vi "ActionVIOnLoad.vi"(8 "error in (no error)":errorcluster, 11 "Device Item Ref in":T1 format="%.0x") -> (0 "error out":errorcluster, 3 "Device Item Ref out":T1 format="%.0x")   [LabVIEW 2019, in "Protection and Counter Addon System Explorer.lvlib"]
uses:
  Protection and Counter Addon System Explorer.lvlib
  <vilib>/NI VeriStand/Custom Device API/Custom Device Item Ref.ctl
  <vilib>/NI VeriStand/Custom Device API/Custom Device Channel.ctl
  <vilib>/NI VeriStand/Custom Device API/Custom Device Channel Type.ctl
  NationalInstruments.VeriStand.SystemDefinitionAPI
  Addon Shared/SubVIs/GUID Lookup.vi
  <vilib>/NI/NI VeriStand Advanced SysDef API/_SubVIs/SysDef.Search.GUID.vi
  <vilib>/NI/NI VeriStand Advanced SysDef API/_SubVIs/SysDef.Search.GUIDs.vi
  <vilib>/NI/NI VeriStand Advanced SysDef API/_SubVIs/SysDef.Search.Parent.vi
  Addon Shared/Protection and Counter Addon Shared.lvlib
  <vilib>/NI/NI VeriStand Advanced SysDef API/SysDef API/Advanced System Definition.lvlib
  <vilib>/NI VeriStand/Custom Device API/Custom Device API.lvlib
  SubModules/Frame-Protection-Support/Source/System Explorer/Protection and Counter Support System Explorer.lvlib
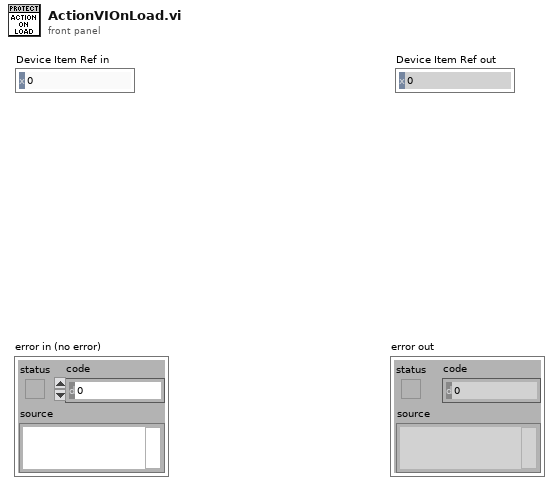
[diagram p1: front panel]
types:
  T1 = typedef "Custom Device API.lvlib/Custom Device Item Ref.ctl" = u64
  T2 = typedef "Custom Device API.lvlib/Custom Device Channel.ctl" = cluster{"Type":T3, "Units":string, "Default Value":dbl, "Faultable":bool, "Scalable":bool}
  T3 = typedef "Custom Device API.lvlib/Custom Device Channel Type.ctl" = enum16{"Input", "Output"}
  T4 = typedef "Protection and Counter Support System Explorer.lvlib/Protection Signal Settings.ctl" = cluster{"Input Channels":T5[], "Protection Type":T6}
  T5 = typedef "Protection and Counter Support System Explorer.lvlib/Protection Signal Linked Channel.ctl" = cluster{"Node Ref":T1}
  T6 = typedef "Protection and Counter Support Shared.lvlib/Protection Type.ctl" = enum16{"Arb ID + Bytes Checksum with Inversion", "Arb ID + Bytes CRC with Inversion", "Reversed Raw Signal Checksum with Inversion", "Concatenated Two's Compliment"}
  T7 = typedef "Advanced System Definition.lvlib/TreeItem.Info.ctl" = cluster{"Name":string, "Description":string, "GUID":string, "Is Channel":bool, "Channel":T2, "Is Waveform":bool, "Waveform":T8}
  T8 = typedef "Custom Device API.lvlib/Custom Device Waveform.ctl" = cluster{"Data Type":T9, "Units":string}
  T9 = typedef "Custom Device API.lvlib/Custom Device Waveform DataType.ctl" = enum16{"Double", "Complex Double"}
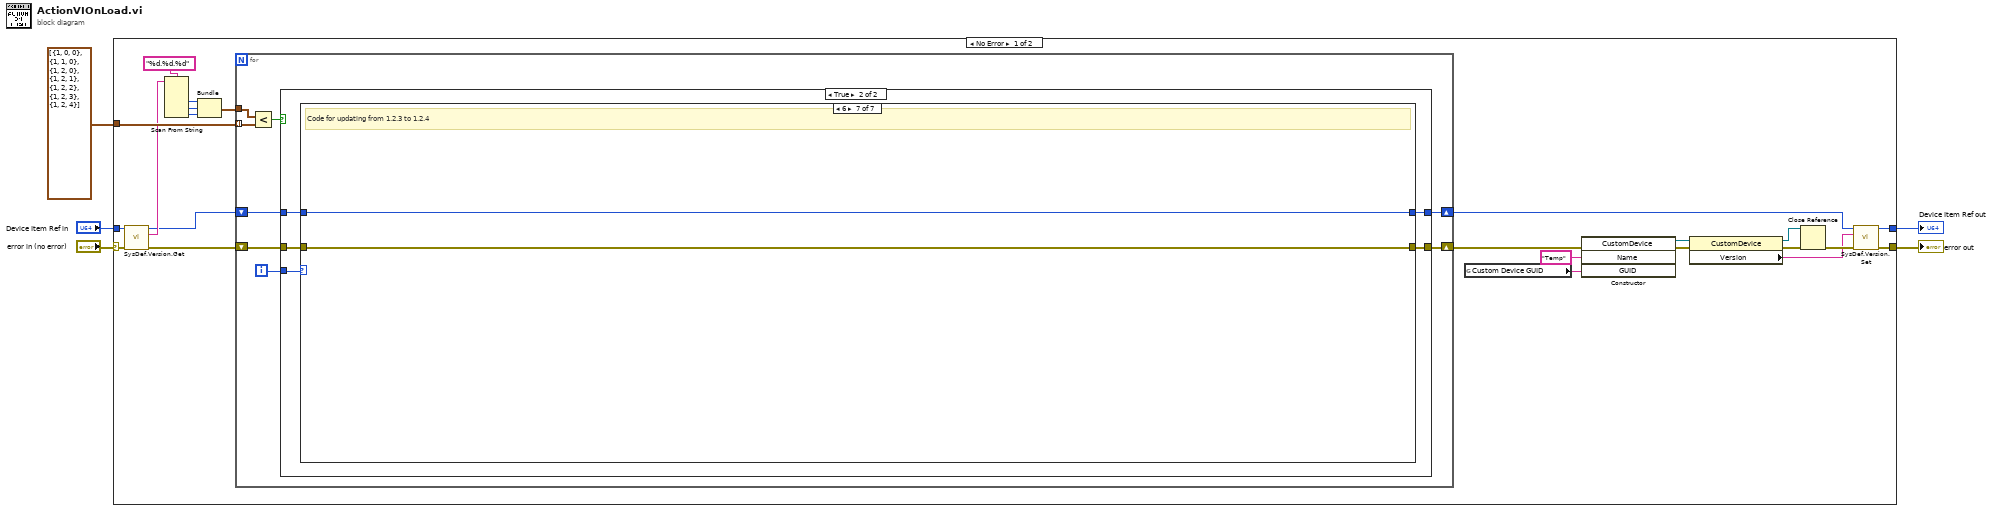
[diagram p0: block diagram]
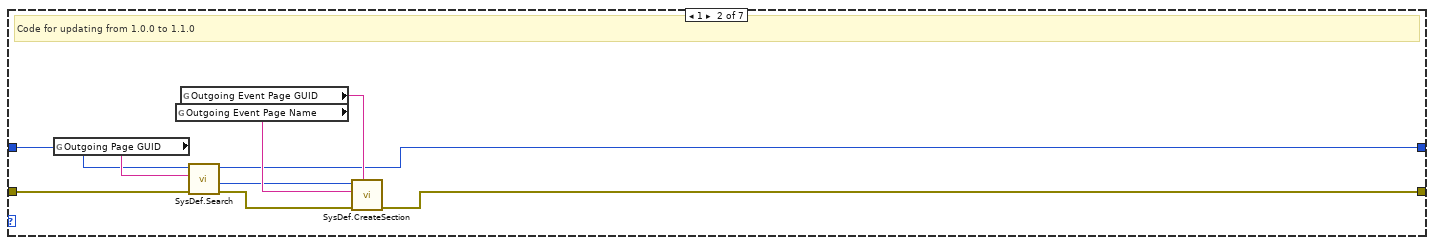
[diagram p4: hidden frame]
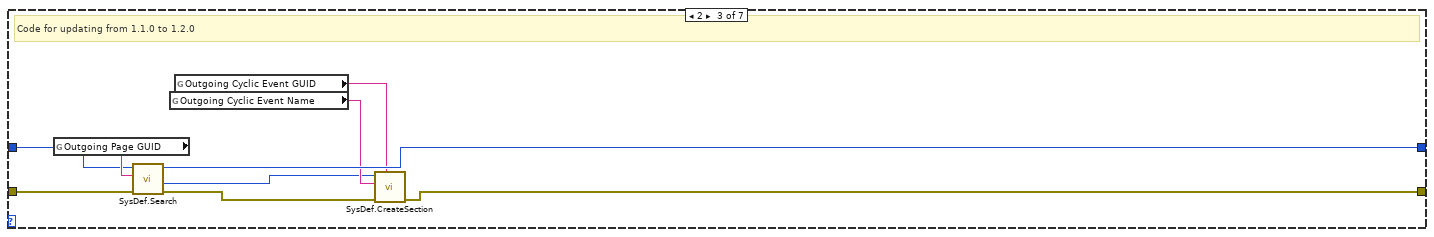
[diagram p5: hidden frame]
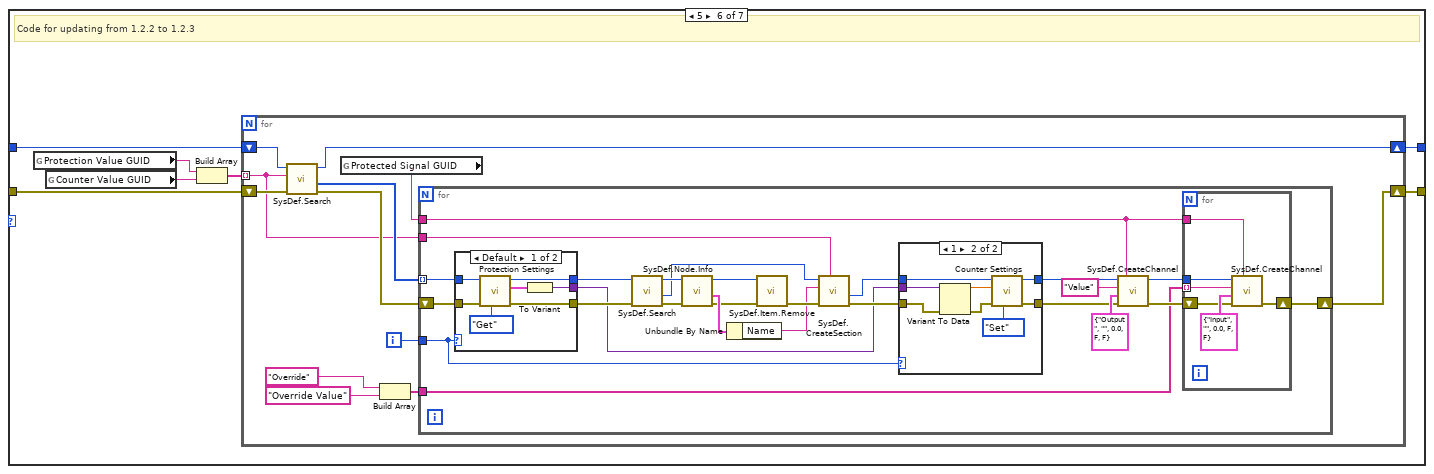
[diagram p8: hidden frame]
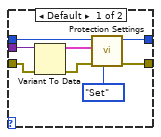
[diagram p9: hidden frame]
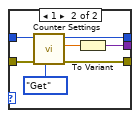
[diagram p10: hidden frame]
diagram:
  n1 = case shown="No Error" "error in (no error)" {
    selector: "error in (no error)" -> [w11 w152]
    tunnel: [w18 w152] -> w4
    tunnel: "Device Item Ref in" -> [w10 w151]
    tunnel: [w16 w151] -> w2
    tunnel: cluster{i32, i32, i32}[] [{1, 0, 0}, {1, 1, 0}, {1, 2, 0}, {1, 2, 1}, {1, 2, 2}, {1, 2, 3}, {1, 2, 4}] -> [w20 _]
    frame No Error {
      n2 = call <vilib>:"SysDef.Version.Get.vi"("error in (no error)"=w11, "nodeID"=w10) -> ("error out"=w7:errorcluster, "Version"=w14:string, "nodeID out"=w6:u64)  [unwired: 7 in]
      n3 = Scan From String(format string="%d.%d.%d", input string=w14) -> (output 1=w13:i32, output 2=w12:i32, output 3=w15:i32)  [unwired: 5 in, 3 out]
      n4 = Bundle(w13, w12, w15) -> (w8:cluster{i32, i32, i32})  [unwired: 1 in]
      n5 = for {
        tunnel: w20 -> [w31] mode=indexing
        shift-right: [w35] -> w19
        shift-left: w7 -> [w29]
        shift-right: [w34] -> w21
        shift-left: w6 -> [w30]
        tunnel: w8 -> [w32]
        i -> [w33]
        n6 = Less?(x=w32, y=w31) -> (x < y?=w36:bool)
        n7 = case shown="True" w36 {
          tunnel: w29 -> [w38 w43]
          tunnel: w30 -> [w37 w42]
          tunnel: [w38 w40] -> w35
          tunnel: [w37 w41] -> w34
          tunnel: w33 -> [_ w39]
          frame False {
          }
          frame True {
            n8 = case shown="6" w39 {
              tunnel: w43 -> [w44 w51 w62 w64 w66 w73 w149]
              tunnel: w42 -> [w45 w50 w61 w65 w67 w68 w150]
              tunnel: [w45 w47 w60 w65 w67 w74 w150] -> w41
              tunnel: [w44 w46 w57 w64 w66 w72 w149] -> w40
              frame Default {
              }
              frame 1 {
                # "Code for updating from 1.0.0 to 1.1.0"
                n9 = global read "GUID Lookup.vi" "Outgoing Page GUID"() -> (w52:string)
                n10 = global read "GUID Lookup.vi" "Outgoing Event Page Name"() -> (w54:string)
                n11 = global read "GUID Lookup.vi" "Outgoing Event Page GUID"() -> (w53:string)
                n12 = call-poly <vilib>:"SysDef.Search.vi"("error in (no error)"=w51, "GUID"=w52, "nodeID"=w50) -> ("error out"=w49:errorcluster, "Value out"=w48:u64, "nodeID out"=w47:u64)  [unwired: 5 in, 1 out]
                n13 = call <vilib>:"SysDef.CreateSection.vi"("GUID"=w53, "error in (no error)"=w49, "Name"=w54, "nodeID"=w48) -> ("error out"=w46:errorcluster)  [unwired: 4 in, 3 out]
              }
              frame 2 {
                # "Code for updating from 1.1.0 to 1.2.0"
                n14 = global read "GUID Lookup.vi" "Outgoing Page GUID"() -> (w63:string)
                n15 = call-poly <vilib>:"SysDef.Search.vi"("error in (no error)"=w62, "GUID"=w63, "nodeID"=w61) -> ("error out"=w56:errorcluster, "Value out"=w55:u64, "nodeID out"=w60:u64)  [unwired: 5 in, 1 out]
                n16 = global read "GUID Lookup.vi" "Outgoing Cyclic Event Name"() -> (w59:string)
                n17 = global read "GUID Lookup.vi" "Outgoing Cyclic Event GUID"() -> (w58:string)
                n18 = call <vilib>:"SysDef.CreateSection.vi"("GUID"=w58, "error in (no error)"=w56, "Name"=w59, "nodeID"=w55) -> ("error out"=w57:errorcluster)  [unwired: 4 in, 3 out]
              }
              frame 3 {
                # "Code for updating from 1.2.0 to 1.2.1"
              }
              frame 4 {
                # "Code for updating from 1.2.1 to 1.2.2"
              }
              frame 5 {
                # "Code for updating from 1.2.2 to 1.2.3"
                n19 = global read "GUID Lookup.vi" "Protection Value GUID"() -> (w71:string)
                n20 = global read "GUID Lookup.vi" "Counter Value GUID"() -> (w70:string)
                n21 = Build Array(w71, w70) -> (w69:string[])
                n22 = for {
                  shift-right: [w86] -> w74
                  shift-left: w68 -> [w85]
                  shift-right: [w81] -> w72
                  shift-left: w73 -> [w84]
                  tunnel: w69 -> [w76] mode=indexing
                  i -> [w75]
                  n23 = call-poly <vilib>:"SysDef.Search.vi"("error in (no error)"=w84, "GUID"=w76, "nodeID"=w85) -> ("error out"=w82:errorcluster, "Values Out"=w83:u64[], "nodeID out"=w86:u64)  [unwired: 5 in, 1 out]
                  n24 = global read "GUID Lookup.vi" "Protected Signal GUID"() -> (w77:string)
                  n25 = Build Array("Override" ("Override Name"), "Override Value" ("Override Value Name")) -> (w78:string[])
                  n26 = for {
                    tunnel: w83 -> [w93] mode=indexing
                    shift-right: [w110] -> w81
                    shift-left: w82 -> [w96]
                    tunnel: w78 -> [w109]
                    tunnel: w77 -> [w107]
                    tunnel: w76 -> [w100]
                    tunnel: w75 -> [w87]
                    n27 = case shown="Default" w87 {
                      tunnel: w96 -> [w133 w141]
                      tunnel: [w132 w140] -> w95
                      tunnel: [w131 w139] -> w94
                      tunnel: w93 -> [w134 w138]
                      tunnel: [w129 w136] -> w88
                      frame Default {
                        n28 = call "Protection Settings.vi"("Action"=enum8{"Get", "Set"}."Get", "error in"=w133, "Parent Ref"=w134) -> ("error out"=w132:errorcluster, "Selected Channels"=w130:T4, "Parent Ref Out"=w131:T1)  [unwired: 6 in]
                        n29 = To Variant(anything=w130) -> (Variant=w129:variant)
                      }
                      frame 1 {
                        n30 = call "Counter Settings.vi"("Action"=enum8{"Get", "Set"}."Get", "error in"=w141, "Parent Ref"=w138) -> ("error out"=w140:errorcluster, "Max Count"=w137:dbl, "Parent Ref Out"=w139:T1)  [unwired: 6 in]
                        n31 = To Variant(anything=w137) -> (Variant=w136:variant)
                      }
                    }
                    n32 = call-poly <vilib>:"SysDef.Search.vi"("error in (no error)"=w95, "nodeID"=w94) -> ("error out"=w99:errorcluster, "Value out"=w97:u64, "nodeID out"=w98:u64)  [unwired: 6 in, 1 out]
                    n33 = call <vilib>:"SysDef.Node.Info.vi"("error in (no error)"=w99, "nodeID"=w98) -> ("error out"=w103:errorcluster, "Item Info"=w105:T7, "nodeID out"=w104:u64)  [unwired: 6 in, 1 out]
                    n34 = Unbundle By Name(w105) -> ("Name"=w101:string)
                    n35 = call <vilib>:"SysDef.Item.Remove.vi"("error in (no error)"=w103, "nodeID"=w104) -> ("error out"=w102:errorcluster)  [unwired: 8 in, 1 out]
                    n36 = call <vilib>:"SysDef.CreateSection.vi"("GUID"=w100, "error in (no error)"=w102, "Name"=w101, "nodeID"=w97) -> ("error out"=w92:errorcluster, "New NodeID"=w90:u64)  [unwired: 4 in, 2 out]
                    n37 = case shown="1" w87 {
                      tunnel: w92 -> [w114 w122]
                      tunnel: [w117 w127] -> w91
                      tunnel: w90 -> [w119 w126]
                      tunnel: [w118 w125] -> w89
                      tunnel: w88 -> [w116 w124]
                      frame Default {
                        n38 = Variant To Data(error in=w114, Variant=w116) -> (data=w113:T4, error out=w115:errorcluster)  [unwired: 1 in]
                        n39 = call "Protection Settings.vi"("Action"=enum8{"Get", "Set"}."Set", "error in"=w115, "Selected Channels"=w113, "Parent Ref"=w119) -> ("error out"=w117:errorcluster, "Parent Ref Out"=w118:T1)  [unwired: 5 in, 1 out]
                      }
                      frame 1 {
                        n40 = Variant To Data(error in=w122, Variant=w124) -> (data=w121:dbl, error out=w123:errorcluster)  [unwired: 1 in]
                        n41 = call "Counter Settings.vi"("Action"=enum8{"Get", "Set"}."Set", "error in"=w123, "Max Count"=w121, "Parent Ref"=w126) -> ("error out"=w127:errorcluster, "Parent Ref Out"=w125:T1)  [unwired: 5 in, 1 out]
                      }
                    }
                    n42 = call <vilib>:"SysDef.CreateChannel.vi"("GUID"=w107, "error in (no error)"=w91, "Channel"=T2 {"Type"=enum."Output", "Units"="", "Default Value"=0.0, "Faultable"=FALSE, "Scalable"=FALSE}, "Name"="Value" ("Override Name"), "nodeID"=w89) -> ("error out"=w111:errorcluster, "nodeID out"=w108:u64)  [unwired: 3 in, 2 out]
                    n43 = for {
                      tunnel: w109 -> [w145] mode=indexing
                      tunnel: w108 -> [w144]
                      tunnel: w107 -> [w143]
                      shift-right: [w146] -> w110
                      shift-left: w111 -> [w147]
                      n44 = call <vilib>:"SysDef.CreateChannel.vi"("GUID"=w143, "error in (no error)"=w147, "Channel"=T2 {"Type"=enum."Input", "Units"="", "Default Value"=0.0, "Faultable"=FALSE, "Scalable"=FALSE}, "Name"=w145, "nodeID"=w144) -> ("error out"=w146:errorcluster)  [unwired: 3 in, 3 out]
                    }
                  }
                }
              }
              frame 6 {
                # "Code for updating from 1.2.3 to 1.2.4"
              }
            }
          }
        }
      }
      n45 = global read "GUID Lookup.vi" "Custom Device GUID"() -> (w17:string)
      n46 = constructor class="CustomDevice"(error in=w19, "Name"="Temp", "GUID"=w17) -> (reference out=w28:refnum<k24>, error out=w27:errorcluster)  [unwired: 2 in, 3 out]
      n47 = property class="CustomDevice"(reference=w28, error in=w27) -> (reference out=w25:refnum<k24>, error out=w26:errorcluster, "Version"=w23:string)
      n48 = Close Reference(reference=w25, error in (no error)=w26) -> (error out=w24:errorcluster)
      n49 = call <vilib>:"SysDef.Version.Set.vi"("error in (no error)"=w24, "Version"=w23, "nodeID"=w21) -> ("error out"=w18:errorcluster, "nodeID out"=w16:u64)  [unwired: 7 in]
    }
    frame Error {
    }
  }
  "error out" <- w4
  "Device Item Ref out" <- w2
